vi "GroveAnalogTestHarness.vi"() -> ()   [LabVIEW 2020, in "CTI-Scratchpad.lvlib"]
uses:
  CTI-Scratchpad.lvlib
  CTI/Identity.ctl
  CTI-Peripheral/Analog Input/Grove An In/I2C/ADC-ADS1115/Private/ConfigData.ctl
  CTI-Peripheral/Analog Input/Grove An In/I2C/ADC-ADS1115/Private/ADS1115Mode.ctl
  CTI-Peripheral/Analog Input/Grove An In/I2C/ADC-ADS1115/Private/ADS1115Mux.ctl
  CTI-Peripheral/Analog Input/Grove An In/I2C/ADC-ADS1115/Private/ADS1115DataRate.ctl
  CTI-Peripheral/Analog Input/Grove An In/I2C/ADC-ADS1115/Private/ADS1115PGA.ctl
  CTI/Error Reporting.ctl
  CTI/GPIO Number.ctl
  CTI/I2C Number.ctl
  CTI/Session/Session.lvclass
  CTI-Peripheral/Analog Input/Grove An In/I2C/ADC-ADS1115/Grove An In ADS1115.lvclass
  CTI-Peripheral/I2C OLED/64x128 I2C OLED SSD1315/64x128 I2C OLED SSD1315.lvclass
  CTI-Peripheral/Analog Output/Grove An Out/M5StackDAC2/M5StackDAC2.lvclass
  CTI/VisaComms/VisaComms.lvclass
  CTI/CTI.lvlib
panel:
  in  "V0":u16(slide)=2000 scale=0.0..32767.0
  in  "V1":u16(slide)=2001 scale=0.0..32767.0
  out "Volts":picture
  in  "Configure ADS1115":T1={"Mode"=enum."Single-Shot", "MUX"=enum."Single AI3 - GND", "Data Rate"=enum."8 SPS", "PGA"=enum."FS = ±6.144V"}
  out "loop":i32
  in  "stop":bool
  out "Identity":T6
  out "error out":errorcluster
  in  "Port":refnum<visa-resource-name>="COM4"
  # "https://wiki.seeedstudio.com/Grove-16-bit-ADC-ADS1115/"
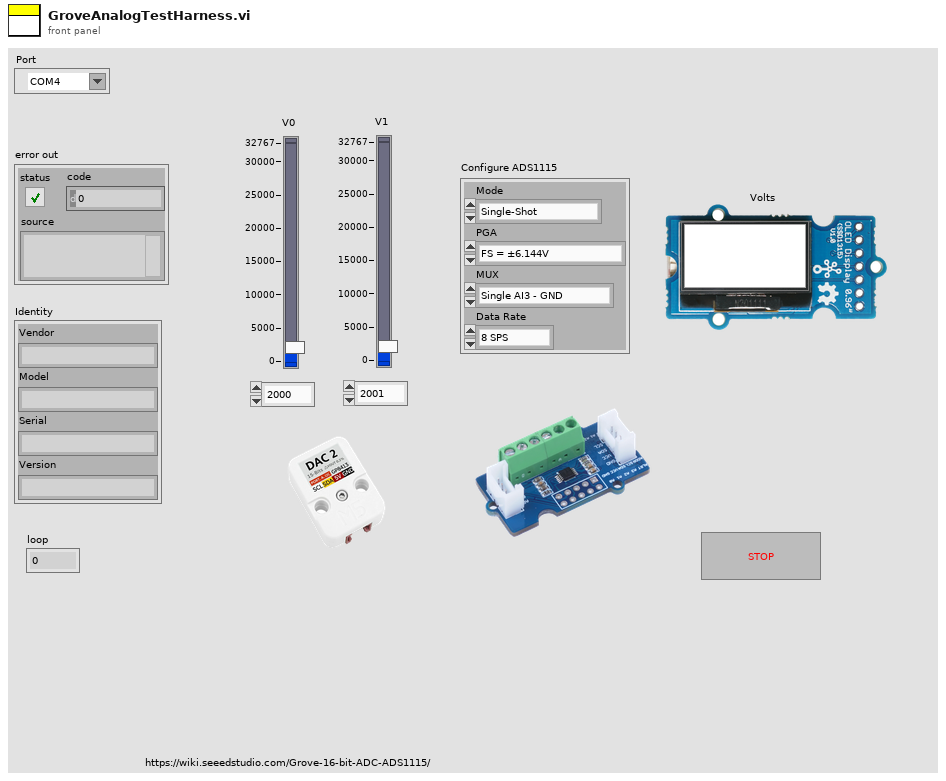
[diagram p1: front panel]
types:
  T1 = typedef "CTI-Peripheral.lvlib/Grove An In ADS1115.lvclass/ConfigData.ctl" = cluster{"Mode":T2, "MUX":T3, "Data Rate":T4, "PGA":T5}
  T2 = typedef "CTI-Peripheral.lvlib/Grove An In ADS1115.lvclass/ADS1115Mode.ctl" = enum16{"Continuous", "Single-Shot"}
  T3 = typedef "CTI-Peripheral.lvlib/Grove An In ADS1115.lvclass/ADS1115Mux.ctl" = enum16{"Single AI0 - GND", "Single AI1 - GND", "Single AI2 - GND", "Single AI3 - GND"}
  T4 = typedef "CTI-Peripheral.lvlib/Grove An In ADS1115.lvclass/ADS1115DataRate.ctl" = enum16{"8 SPS", "16 SPS", "32 SPS", "64 SPS", "128 SPS", "250 SPS", "475 SPS", "860 SPS"}
  T5 = typedef "CTI-Peripheral.lvlib/Grove An In ADS1115.lvclass/ADS1115PGA.ctl" = enum16{"FS = ±6.144V", "FS = ±4.096V", "FS = ±2.048V", "FS = ±1.024V", "FS = ±0.512V", "FS = ±0.256V"}
  T6 = typedef "CTI.lvlib/Identity.ctl" = cluster{"Vendor":string, "Model":string, "Serial":string, "Version":string}
  T7 = typedef "CTI.lvlib/GPIO Number.ctl" = i8
  T8 = typedef "CTI.lvlib/I2C Number.ctl" = i8
  T9 = typedef "CTI.lvlib/Error Reporting.ctl" = enum16{"Minimal", "Moderate", "Full"}
  T10 = enum16{"User-specified Font", "Application Font", "System Font", "Dialog Font"}
  T11 = cluster{"horizontal":enum16{"left", "center", "right"}, "vertical":enum16{"top", "center", "bottom"}}
  T12 = cluster{"Font Name:":string, "Size":i16, "Strikeout?":bool, "Italic?":bool, "Underline?":bool, "Outline?":bool, "Shadow?":bool, "Bold?":bool}
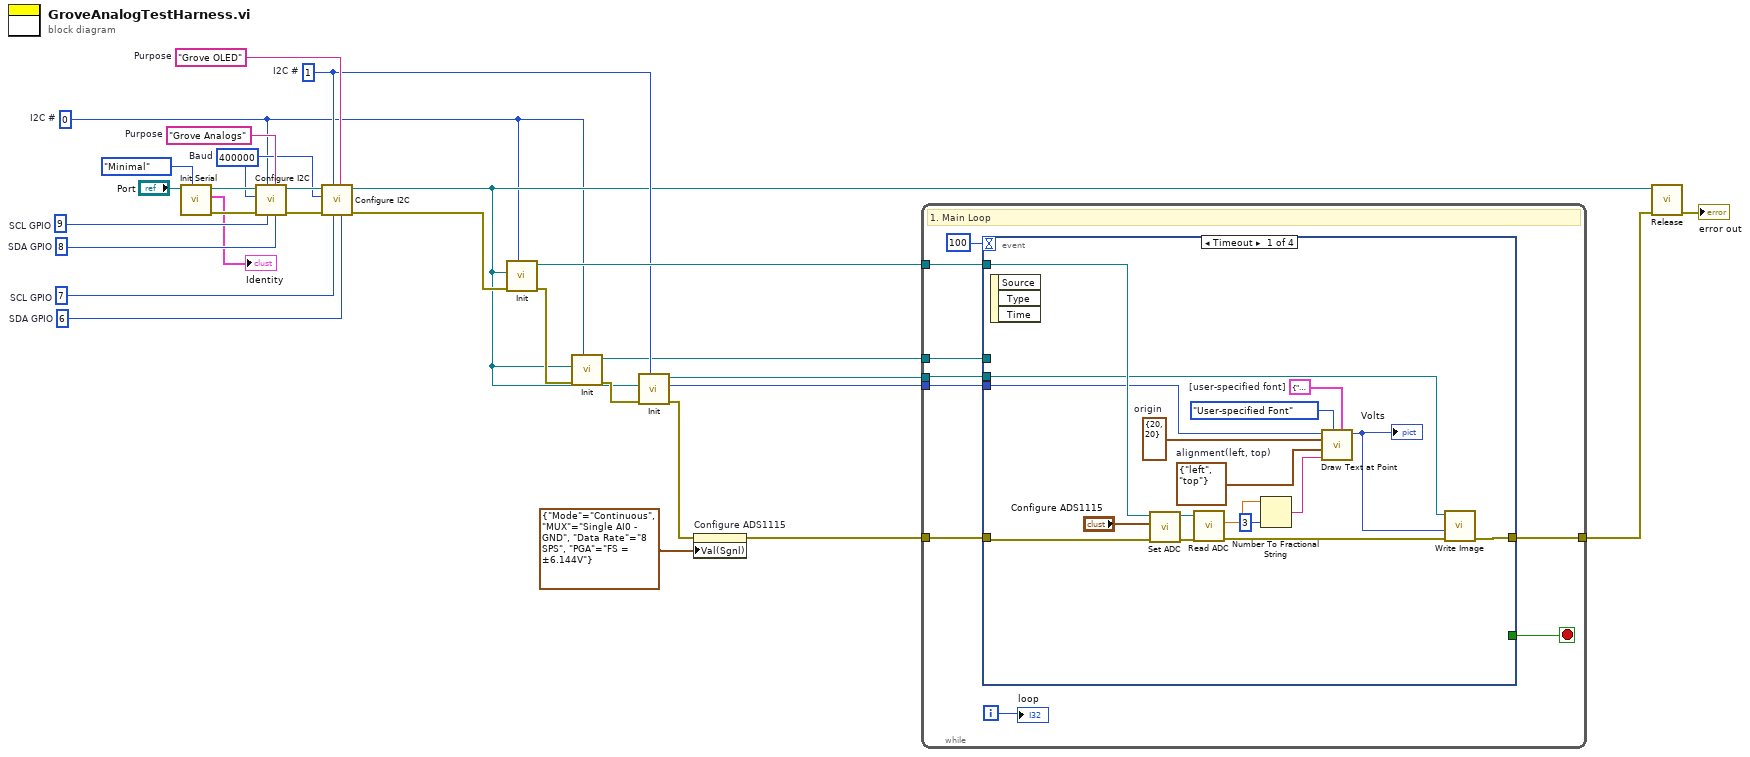
[diagram p0: block diagram]
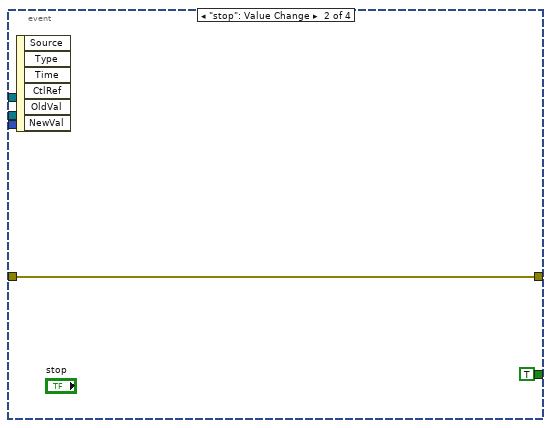
[diagram p2: hidden frame]
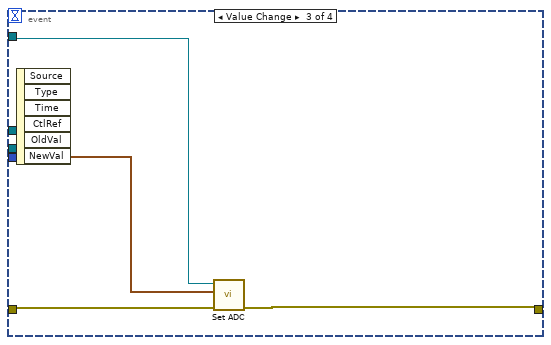
[diagram p3: hidden frame]
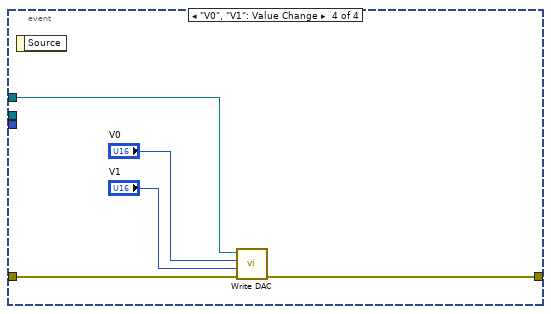
[diagram p4: hidden frame]
diagram:
  w12 = T7 6  # SDA GPIO
  w13 = T7 7  # SCL GPIO
  w14 = "Grove OLED"  # Purpose
  w10 = T8 1  # I2C #
  w1 = T8 0  # I2C #
  w23 = T7 8  # SDA GPIO
  w24 = T7 9  # SCL GPIO
  w25 = "Grove Analogs"  # Purpose
  w15 = u32 400000  # Baud
  n1 = call "Init Serial.vi"("Error Checking (Full)"=Error_Reporting."Minimal", "VISA resource name in"="Port") -> ("error out"=w26:errorcluster, "Identity"=→"Identity":T6, "Session"=w27:refnum<class "Session.lvclass">)  [unwired: 7 in]
  n2 = call "Configure I2C.vi"("SDA GPIO"=w23, "Purpose (\"I2C\")"=w25, "SCL GPIO"=w24, "I2C #"=w1, "error in (no error)"=w26, "Baud"=w15, "Session in"=w27) -> ("error out"=w17:errorcluster, "Session out"=w16:refnum<class "Session.lvclass">)  [unwired: 3 in]
  n3 = call "Configure I2C.vi"("SDA GPIO"=w12, "Purpose (\"I2C\")"=w14, "SCL GPIO"=w13, "I2C #"=w10, "error in (no error)"=w17, "Baud"=w15, "Session in"=w16) -> ("error out"=w11:errorcluster, "Session out"=w2:refnum<class "Session.lvclass">)  [unwired: 3 in]
  n4 = call "Init.vi"("I2C #"=w1, "error in (no error)"=w11, "Session In"=w2) -> ("error out"=w5:errorcluster, "ADS115 Out"=w21:refnum<class "Grove An In ADS1115.lvclass">)  [unwired: 7 in]
  n5 = call "Init.vi"("I2C #"=w1, "error in (no error)"=w5, "Session In"=w2) -> ("error out"=w4:errorcluster, "M5StackDAC2 Out"=w3:refnum<class "M5StackDAC2.lvclass">)  [unwired: 7 in]
  n6 = call "Init.vi"("I2C #"=w10, "error in (no error)"=w4, "Session In"=w2) -> ("error out"=w8:errorcluster, "2D Picture"=w7:picture, "64x128 I2C OLED SSD1315 Out"=w9:refnum<class "64x128 I2C OLED SSD1315.lvclass">)  [unwired: 6 in]
  n7 = property on="Configure ADS1115" class="Clust (strict)"(error in=w8, "Val(Sgnl)"=T1 {"Mode"=enum."Continuous", "MUX"=enum."Single AI0 - GND", "Data Rate"=enum."8 SPS", "PGA"=enum."FS = ±6.144V"} ("Value (Signaling)")) -> (error out=w6:errorcluster)  [unwired: 1 in, 1 out]
  n8 = while {
    tunnel: w6 -> [w37]
    tunnel: w21 -> [w38]
    tunnel: [w35] -> w20
    tunnel: w9 -> [w31]
    tunnel: w7 -> [w32]
    tunnel: w3 -> [w30]
    i -> [w36]
    stop <- w33 stop-if-true
    # "1. Main Loop"
    n9 = event shown="[0] Timeout" {
      selector: _ -> [_ _ _ _]
      dyn-events: _ -> [_ _ _ _]
      timeout: 100 -> [_ _ _ _]
      tunnel: w38 -> [w54 _ w59 _]
      tunnel: w37 -> [w53 w56 w61 w63]
      tunnel: [w48 w56 w58 w62] -> w35
      tunnel: [_ TRUE _ _] -> w33
      tunnel: w32 -> [w50 _ _ _]
      tunnel: w31 -> [w45 _ _ _]
      tunnel: w30 -> [_ _ _ w64]
      event Timeout {
        w40 = T11 {"horizontal"=enum."left", "vertical"=enum."top"}  # alignment(left, top)
        w41 = cluster{"x":i16, "y":i16} {"x"=20, "y"=20}  # origin
        w39 = T12 {"Font Name:"="Courier New", "Size"=32, "Strikeout?"=FALSE, "Italic?"=FALSE, "Underline?"=FALSE, "Outline?"=FALSE, "Shadow?"=FALSE, "Bold?"=TRUE}  # [user-specified font]
        n10 = event-data() -> ()  [unwired: 1 in, 3 out]
        n11 = call-dynamic "Set ADC.vi"("error in (no error)"=w53, "Configure ADS1115"="Configure ADS1115", "ADS1115 in"=w54) -> ("error out"=w51:errorcluster, "ADS1115 out"=w55:refnum<class "Grove An In ADS1115.lvclass">)  [unwired: 7 in]
        n12 = call-dynamic "Read ADC.vi"("error in (no error)"=w51, "ADS1115 in"=w55) -> ("error out"=w49:errorcluster, "Data Out"=w44:dbl)  [unwired: 7 in, 1 out]
        n13 = Number To Fractional String(number=w44, precision (6)=i16 3) -> (F-format string=w42:string)  [unwired: 2 in]
        n14 = call <vilib>:"Draw Text at Point.vi"("[user-specified font]"=w39, "desired font(Application)"=T10."User-specified Font", "text"=w42, "alignment(left, top)"=w40, "origin"=w41, "picture"=w50) -> ("new picture"=w46:picture)  [unwired: 4 in, 1 out]
        "Volts" <- w46
        n15 = call-dynamic "Write Image.vi"("error in (no error)"=w49, "2D Picture"=w46, "64x128 I2C OLED SSD1315 In"=w45) -> ("error out"=w48:errorcluster)  [unwired: 7 in, 1 out]
      }
      event "stop": Value Change {
        n16 = event-data() -> ()  [unwired: 1 in, 6 out]
      }
      event Value Change {
        n17 = event-data() -> ("NewVal"=w60:T1)  [unwired: 1 in, 5 out]
        n18 = call-dynamic "Set ADC.vi"("error in (no error)"=w61, "Configure ADS1115"=w60, "ADS1115 in"=w59) -> ("error out"=w58:errorcluster)  [unwired: 7 in, 1 out]
      }
      event "V0", "V1": Value Change {
        n19 = event-data() -> ()  [unwired: 1 in, 1 out]
        n20 = call-dynamic "Write DAC.vi"("error in (no error)"=w63, "Analog Output V1"="V1", "Analog Output VO"="V0", "M5StackDAC2 in"=w64) -> ("error out"=w62:errorcluster)  [unwired: 6 in, 1 out]
      }
    }
    "loop" <- w36
  }
  n21 = call-dynamic "Release.vi"("error in (no error)"=w20, "Session in"=w2) -> ("error out"=→"error out":errorcluster)  [unwired: 9 in]
